vi "Logging Message Loop.vi"(8 "error in (no error)":errorcluster, 10 "Data Queue":refnum<queue>, 11 "Message Queues":T1) -> (0 "error out":errorcluster)   [LabVIEW 2022 SP3, in "Logging.lvlib"]
doc: "The message loop subVI to handle messages pertaining to logging data."
uses:
  Logging.lvlib
  support/Message Queue/All Message Queues.ctl
  support/Message Queue/Message Cluster.ctl
  Logging Configuration.ctl
  Logging State.ctl
  support/Message Queue/Enqueue Message (Single).vi
  <vilib>/Utility/error.llb/Error Cluster From Error Code.vi
  <vilib>/ErrorRing/Error Ring.xnode
  support/Message Queue/Message Queue.lvlib
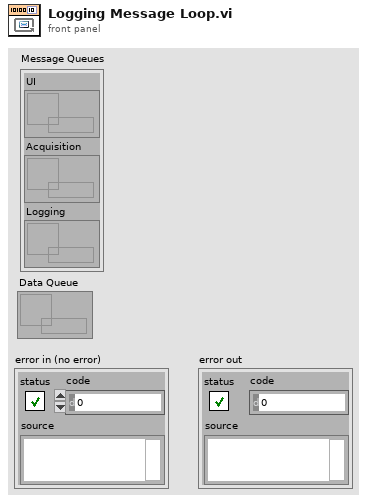
[diagram p1: front panel]
types:
  T1 = typedef "Message Queue.lvlib/All Message Queues.ctl" = cluster{"UI":refnum<queue>, "Acquisition":refnum<queue>, "Logging":refnum<queue>}
  T2 = typedef "Logging.lvlib/Logging Configuration.ctl" = cluster{"TDMS File Reference":refnum<k34>, "Log File Base Path":path}
  T3 = typedef "Logging.lvlib/Logging State.ctl" = enum16{"Idle", "Logging"}
  T4 = enum16{"open", "open or create", "create or replace", "create", "open (read-only)"}
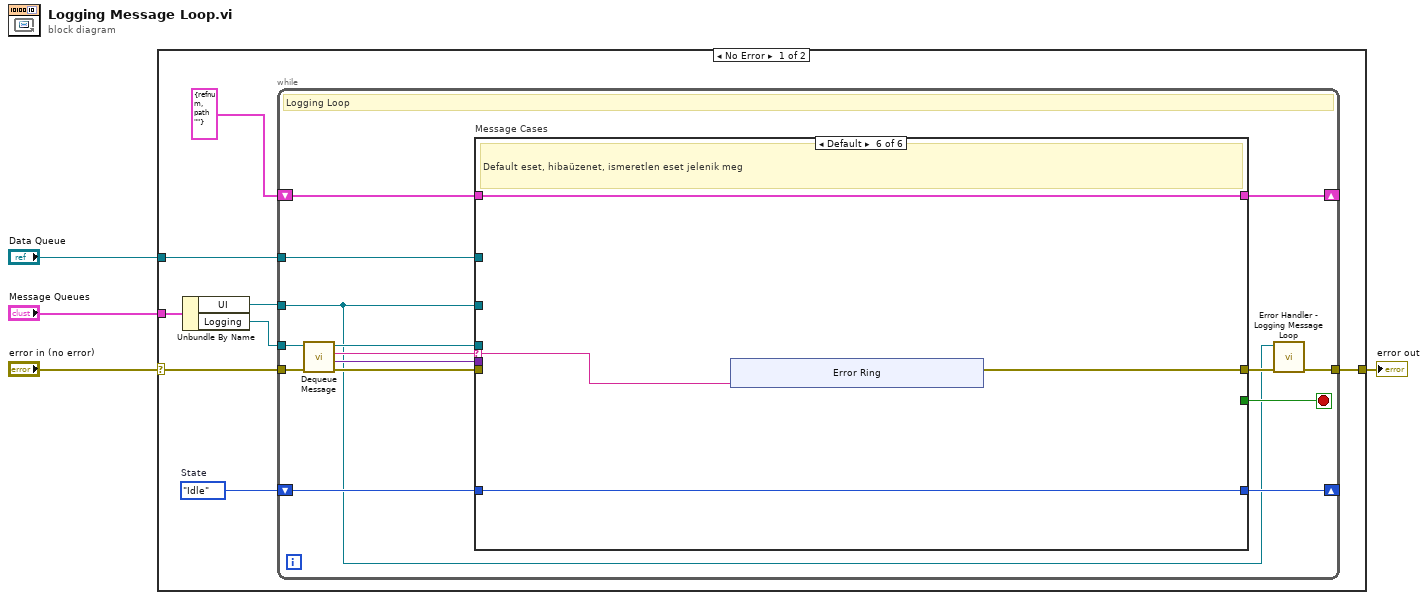
[diagram p0: block diagram]
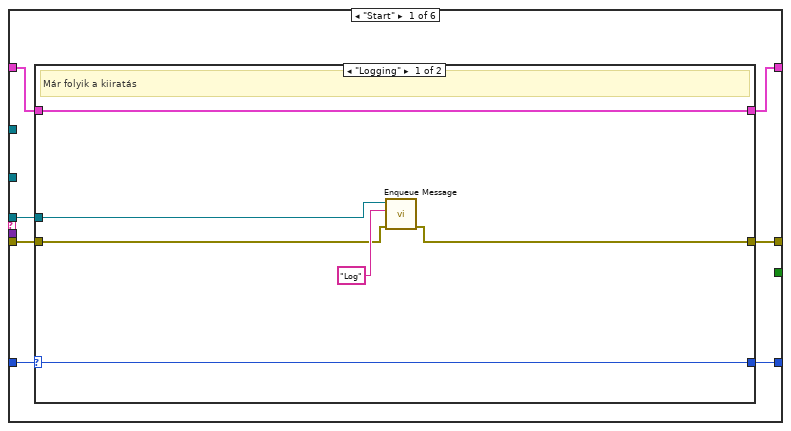
[diagram p2: hidden frame]
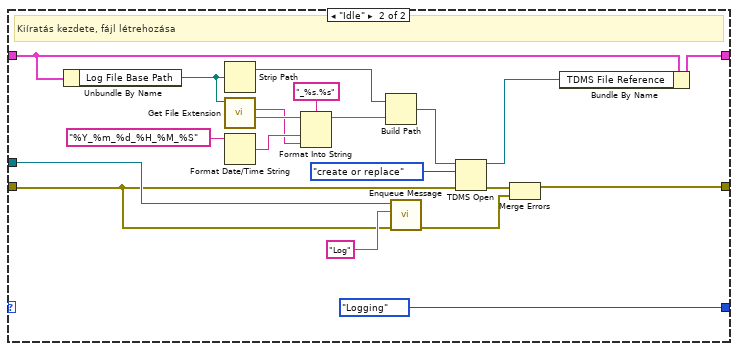
[diagram p3: hidden frame]
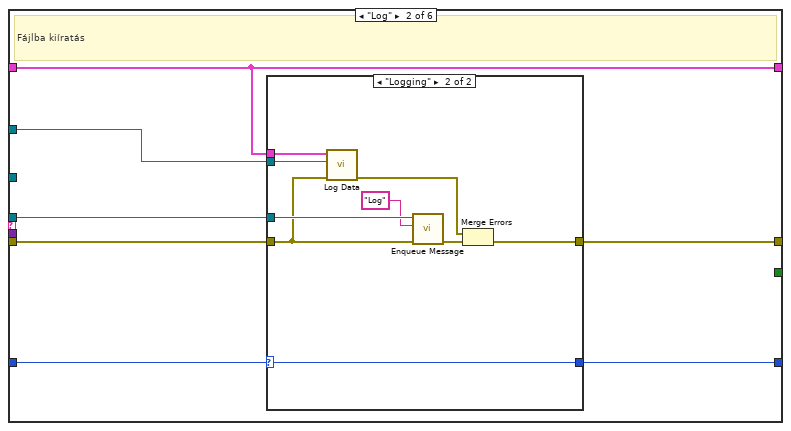
[diagram p4: hidden frame]
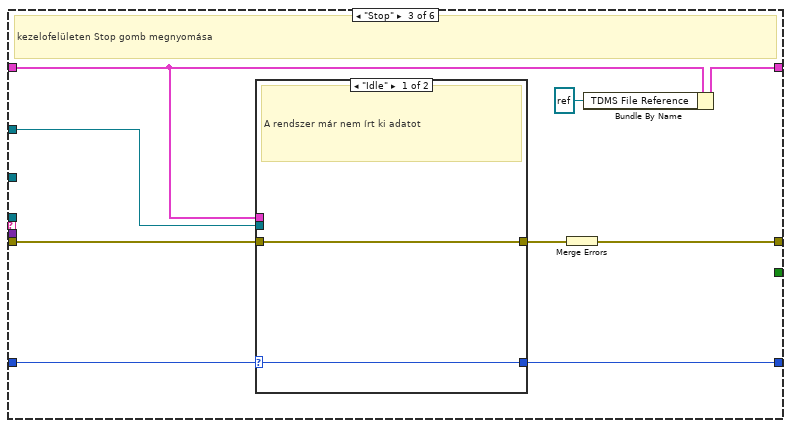
[diagram p6: hidden frame]
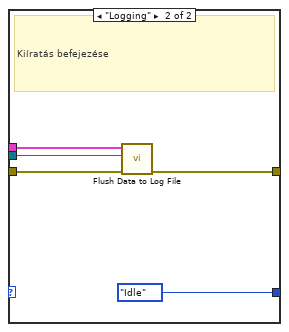
[diagram p7: hidden frame]
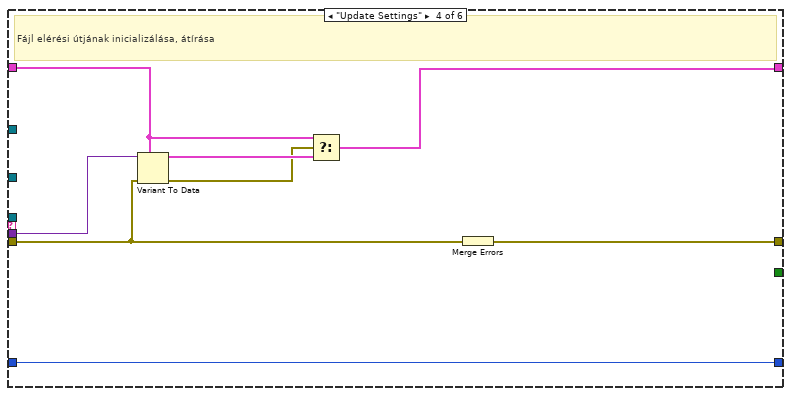
[diagram p8: hidden frame]
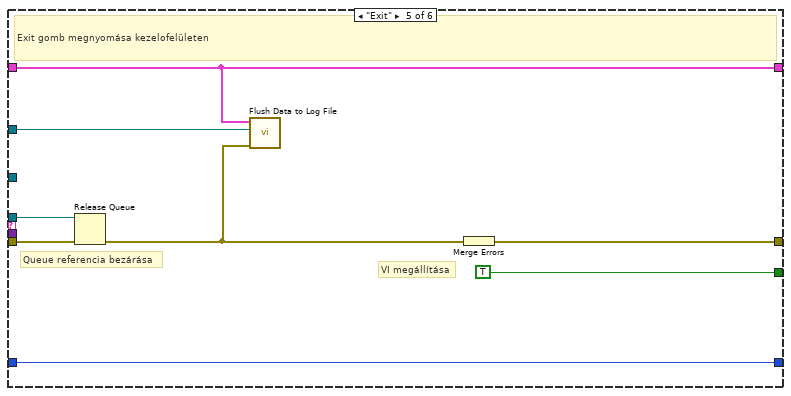
[diagram p9: hidden frame]
diagram:
  n1 = case shown="No Error" "error in (no error)" {
    selector: "error in (no error)" -> [w8 w122]
    tunnel: "Message Queues" -> [w12 _]
    tunnel: [w10 w122] -> w3
    tunnel: "Data Queue" -> [w7 _]
    frame No Error {
      w5 = Logging_State."Idle"  # State
      n2 = Unbundle By Name(w12) -> ("UI"=w6:refnum<queue>, "Logging"=w11:refnum<queue>)
      n3 = while {
        tunnel: w11 -> [w19]
        shift-right: [w26] -> _
        shift-left: T2 {"TDMS File Reference"=refnum, "Log File Base Path"=path ""} ("Logging Configuration") -> [w27]
        tunnel: w6 -> [w13]
        tunnel: w7 -> [w18]
        shift-right: [w16] -> _
        shift-left: w5 -> [w17]
        tunnel: w8 -> [w24]
        tunnel: [w15] -> w10
        stop <- w25 stop-if-true
        # "Logging Loop"
        n4 = call "Dequeue Message.vi"("error in (no error)"=w24, "Message Queue"=w19) -> ("error out"=w23:errorcluster, "Message Data"=w21:variant, "Message"=w22:string, "dup Message Queue"=w20:refnum<queue>)  [unwired: 6 in]
        n5 = case "Message Cases" shown="Default" w22 {
          selector: w22 -> [_ _ _ _ _ w111]
          tunnel: w20 -> [w33 w66 _ _ w107 _]
          tunnel: w23 -> [w32 w64 w81 w96 w108 _]
          tunnel: [w34 w67 w87 w102 w109 w112] -> w14
          tunnel: w27 -> [w31 w63 w82 w100 w105 w114]
          tunnel: [w30 w63 w85 w97 w105 w114] -> w26
          tunnel: [_ _ _ _ TRUE _] -> w25
          tunnel: w21 -> [_ _ _ w101 _ _]
          tunnel: w13 -> [_ _ _ _ _ _]
          tunnel: w18 -> [_ w65 w83 _ w104 _]
          tunnel: w17 -> [w29 w62 w80 w95 w103 w113]
          tunnel: [w28 w61 w79 w95 w103 w113] -> w16
          frame "Start" {
            n6 = case shown="\"Logging\"" w29 {
              selector: w29 -> [w39 _]
              tunnel: [w36 w42] -> w34
              tunnel: w33 -> [w38 w43]
              tunnel: w32 -> [w35 w41]
              tunnel: w31 -> [w40 w44]
              tunnel: [w40 w46] -> w30
              tunnel: [w39 Logging_State."Logging" ("State")] -> w28
              frame "Logging" {
                # "Már folyik a kiiratás"
                n7 = call-poly "Enqueue Message.vi"("error in (no error)"=w35, "Message"="Log", "Message Queue"=w38) -> ("error out"=w36:errorcluster)  [unwired: 7 in, 1 out]
              }
              frame "Idle" {
                # "Kiíratás kezdete, fájl létrehozása"
                n8 = Unbundle By Name(w44) -> ("Log File Base Path"=w59:path)
                n9 = Strip Path(path=w59) -> (stripped path=w56:path)  [unwired: 1 out]
                n10 = call <vilib>:"Get File Extension.vi"("file"=w59) -> ("filename without extension"=w57:string, "lowercase file extension"=w53:string)  [unwired: 6 in, 3 out]
                n11 = Format Date/Time String(time format string (%c)="%Y_%m_%d_%H_%M_%S") -> (date/time string=w54:string)  [unwired: 2 in]
                n12 = Format Into String(format string="_%s.%s", initial string=w57, w54, w53) -> (resulting string=w52:string)  [unwired: 1 in, 1 out]
                n13 = Build Path(base path=w56, name or relative path=w52) -> (appended path=w51:path)
                n14 = call-poly "Enqueue Message.vi"("error in (no error)"=w41, "Message"="Log", "Message Queue"=w43) -> ("error out"=w49:errorcluster)  [unwired: 7 in, 1 out]
                n15 = TDMS Open(8:w41, 10:T4."create or replace" ("operation (0:open)"), 11:w51) -> (0:w50:errorcluster, 3:w47:refnum<k34>)  [unwired: 4 in]
                n16 = Merge Errors(w50, w49) -> (w42:errorcluster)
                n17 = Bundle By Name(cluster=w44, "TDMS File Reference"=w47) -> (w46:T2)
              }
            }
          }
          frame "Log" {
            # "Fájlba kiíratás"
            n18 = case shown="\"Logging\"" w62 {
              selector: w62 -> [w69 w71]
              tunnel: [w68 w78] -> w67
              tunnel: w66 -> [_ w76]
              tunnel: w65 -> [_ w75]
              tunnel: w64 -> [w68 w70]
              tunnel: w63 -> [_ w72]
              tunnel: [w69 w71] -> w61
              frame "Idle" {
              }
              frame "Logging" {
                n19 = call "Log Data.vi"("error in (no error)"=w70, "Data Queue"=w75, "Logging Configuration"=w72) -> ("error out"=w74:errorcluster)  [unwired: 8 in]
                n20 = call-poly "Enqueue Message.vi"("error in (no error)"=w70, "Message"="Log", "Message Queue"=w76) -> ("error out"=w77:errorcluster)  [unwired: 7 in, 1 out]
                n21 = Merge Errors(w74, w77) -> (w78:errorcluster)
              }
            }
          }
          frame "Stop" {
            # "kezelofelületen Stop gomb megnyomása"
            n22 = case shown="\"Idle\"" w80 {
              selector: w80 -> [w88 _]
              tunnel: [w89 w90] -> w86
              tunnel: w83 -> [_ w94]
              tunnel: w82 -> [_ w93]
              tunnel: w81 -> [w89 w92]
              tunnel: [w88 Logging_State."Idle" ("State")] -> w79
              frame "Idle" {
                # "A rendszer már nem írt ki adatot"
              }
              frame "Logging" {
                # "Kiíratás befejezése"
                n23 = call "Flush Data to Log File.vi"("error in (no error)"=w92, "Data Queue"=w94, "Logging Configuration"=w93) -> ("error out"=w90:errorcluster)  [unwired: 8 in]
              }
            }
            n24 = Merge Errors(w86) -> (w87:errorcluster)
            n25 = Bundle By Name(cluster=w82, "TDMS File Reference"=refnum<k34> refnum) -> (w85:T2)
          }
          frame "Update Settings" {
            # "Fájl elérési útjának inicializálása, átírása"
            n26 = Variant To Data(error in=w96, type=w100, Variant=w101) -> (data=w99:T2, error out=w98:errorcluster)
            n27 = Select(t=w100, s=w98, f=w99) -> (s? t:f=w97:T2)
            n28 = Merge Errors(w96) -> (w102:errorcluster)
          }
          frame "Exit" {
            # "Queue referencia bezárása"
            # "VI megállítása"
            # "Exit gomb megnyomása kezelofelületen"
            n29 = Release Queue(queue=w107, error in (no error)=w108) -> (error out=w106:errorcluster)  [unwired: 1 in, 2 out]
            n30 = call "Flush Data to Log File.vi"("error in (no error)"=w106, "Data Queue"=w104, "Logging Configuration"=w105) -> ()  [unwired: 8 in, 1 out]
            n31 = Merge Errors(w106) -> (w109:errorcluster)
          }
          frame Default {
            # "Default eset, hibaüzenet, ismeretlen eset jelenik meg"
            n32 = xnode "Error Ring"("parameter 0"=w111) -> ("error out"=w112:errorcluster)
          }
        }
        n33 = call "Error Handler - Logging Message Loop.vi"("error in (no error)"=w14, "Message Queue"=w13) -> ("dup error in"=w15:errorcluster)  [unwired: 8 in, 1 out]
      }
    }
    frame Error {
    }
  }
  "error out" <- w3
